vi "Write FPPos.vi"(3 "FP":refnum<class "DecFrame_FP.lvclass">, 4 "Position":refnum<class "Frame_FPPos.lvclass">) -> (5 "FP Out":refnum<class "DecFrame_FP.lvclass">)   [LabVIEW 2020, in "DecFrame_FP.lvclass"]
uses:
  DecFrame_FP/DecFrame_FP.lvclass
  Frame_FPPos/Frame_FPPos.lvclass
  DecFrame_FP/DecFrame_FP.lvclass/DecFrame_FP.ctl
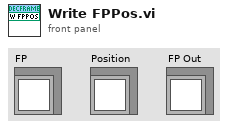
[diagram p1: front panel]
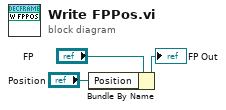
[diagram p0: block diagram]
diagram:
  n1 = Bundle By Name(cluster="FP", "Position"="Position") -> (→"FP Out":refnum<class "DecFrame_FP.lvclass">)
